vi "Write tcp timeouts.vi"(8 "error in (no error)":errorcluster, 10 "tcp timeouts":T1={"connect timeout"=60000, "write timeout"=10000, "read timeout"=10000}, 11 "MB_TCP in":refnum<class "MB_TCP.lvclass">) -> (0 "error out":errorcluster, 3 "MB_TCP out":refnum<class "MB_TCP.lvclass">)   [LabVIEW 2019, in "MB_TCP.lvclass"]
uses:
  MB_TCP.lvclass
  NI_modbus_upd/TCP/tcp timeouts.ctl
  MB_TCP.lvclass/MB_TCP.ctl
  NI_modbus_upd/TCP/TCP.lvclass/TCP.ctl
  NI_modbus_upd/TCP/TCP.lvclass
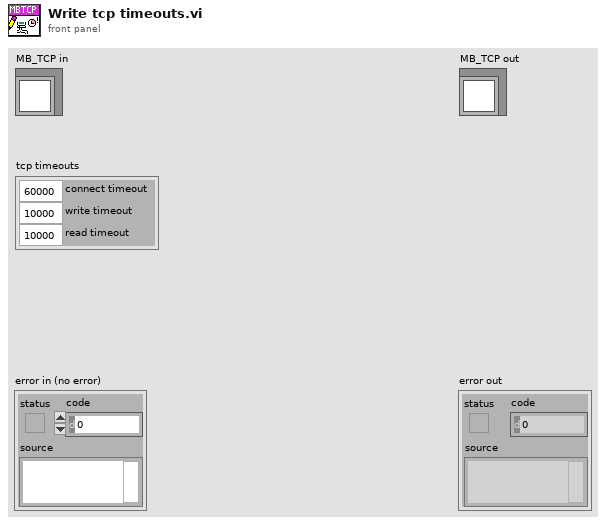
[diagram p1: front panel]
types:
  T1 = typedef "TCP.lvclass/tcp timeouts.ctl" = cluster{"connect timeout":i32, "write timeout":i32, "read timeout":i32}
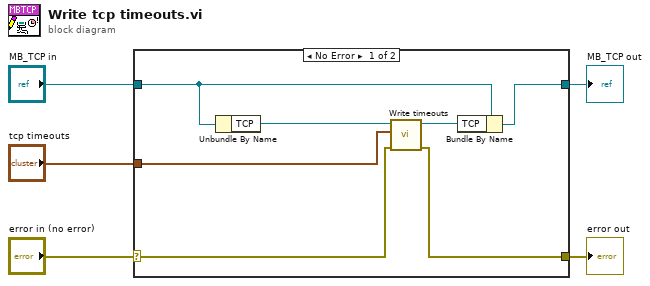
[diagram p0: block diagram]
diagram:
  n1 = case shown="No Error" "error in (no error)" {
    selector: "error in (no error)" -> [w9 w13]
    tunnel: [w8 w13] -> w4
    tunnel: [w12 w14] -> w2
    tunnel: "MB_TCP in" -> [w10 w14]
    tunnel: "tcp timeouts" -> [w6 _]
    frame No Error {
      n2 = Unbundle By Name(w10) -> ("TCP"=w7:refnum<class "TCP.lvclass">)
      n3 = call "Write timeouts.vi"("error in (no error)"=w9, "timeouts"=w6, "TCP Master in"=w7) -> ("error out"=w8:errorcluster, "TCP Master out"=w11:refnum<class "TCP.lvclass">)  [unwired: 7 in]
      n4 = Bundle By Name(cluster=w10, "TCP"=w11) -> (w12:refnum<class "MB_TCP.lvclass">)
    }
    frame Error {
    }
  }
  "error out" <- w4
  "MB_TCP out" <- w2
